vi "NewAutoDashRead.vi"() -> (0 "P3":dbl, 1 "P2":dbl, 2 "P1":dbl, 3 "Timeout":dbl, 4 "StepString":string, 5 "StepType":T1, 7 "StepIndex":i64)   [LabVIEW 2023]
uses:
  <vilib>/Rock Robotics/WPI/ThirdParty/JAS_Junk/TrajLib/VI/BoolCmd_Send.vi
  Wrist/WristCancelSendCmd.vi
  <vilib>/Rock Robotics/WPI/ThirdParty/JAS_Junk/TrajLib/VI/BoolCmd_Send_Internal.vi
  <vilib>/Rock Robotics/WPI/ThirdParty/JAS_Junk/TrajLib/VI/BoolCmd_ObtainQueue.vi
  <vilib>/Rock Robotics/Network Tables/NT Read Integer.vi
  <vilib>/Rock Robotics/Network Tables/NT Read Number.vi
  <vilib>/Rock Robotics/Network Tables/NT Read String.vi
  NewAutoStepTypeEnum.ctl
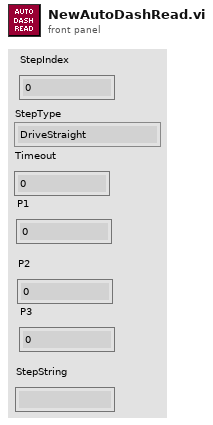
[diagram p1: front panel]
types:
  T1 = typedef "NewAutoStepTypeEnum.ctl" = enum16{"DriveStraight", "DriveTurn", "FollowAbsoluteTrajectory", "FollowRelativeTrajectory", "AutoWait", "ElevToRest", "ElevToFloor", "ElevToSource", "ElevToL1", "ElevToL2", "ElevToL3", "ElevToL4", "ElevToAlgae1", "ElevToAlgae2", "ElevToBarge", "ElevCancel", "IntakeCoral", "IntakeAlgae", "IntakeDepositCoral", "IntakeDepositAlgae", "IntakeCancel", "ElevRestWait", "ElevFloorWait", "ElevSourceWait", "ElevL1Wait", "ElevL2Wait", "ElevAlgae1Wait", "ElevL3Wait", "ElevAlgae2Wait", "ElevL4Wait", "ElevBargeWait", "IntakeWait", "FollowAbsTrajWithTimedCmd", "FollowRelTrajWithTimedCmd"}
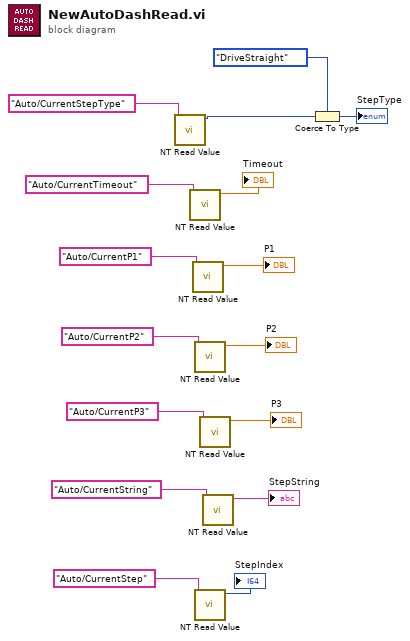
[diagram p0: block diagram]
diagram:
  n1 = call-poly <vilib>:"NT Read Value.vi"("name"="Auto/CurrentStepType") -> ("value"=w8:i64)  [unwired: 8 in, 2 out]
  n2 = call-poly <vilib>:"NT Read Value.vi"("name"="Auto/CurrentTimeout") -> ("value"=→"Timeout":dbl)  [unwired: 8 in, 2 out]
  n3 = call-poly <vilib>:"NT Read Value.vi"("name"="Auto/CurrentP1") -> ("value"=→"P1":dbl)  [unwired: 8 in, 2 out]
  n4 = call-poly <vilib>:"NT Read Value.vi"("name"="Auto/CurrentP2") -> ("value"=→"P2":dbl)  [unwired: 8 in, 2 out]
  n5 = call-poly <vilib>:"NT Read Value.vi"("name"="Auto/CurrentStep") -> ("value"=→"StepIndex":i64)  [unwired: 8 in, 2 out]
  n6 = call-poly <vilib>:"NT Read Value.vi"("name"="Auto/CurrentP3") -> ("value"=→"P3":dbl)  [unwired: 8 in, 2 out]
  n7 = call-poly <vilib>:"NT Read Value.vi"("name"="Auto/CurrentString") -> ("value"=→"StepString":string)  [unwired: 8 in, 2 out]
  n8 = Coerce To Type(0:w8, 1:NewAutoStepTypeEnum."DriveStraight" ("Function")) -> (2:→"StepType":T1)
